vi "FTP Get File List.vi"(8 "에러 입력(에러 없음)":errorcluster, 11 "remote path":string) -> (0 "에러 출력":errorcluster, 1 "remote File path":string[](array[string]), 2 "File List":T1(array[cluster]), 4 "data":string)   [LabVIEW 2020]
uses:
  <vilib>/FTP/NI_FTP.lvlib
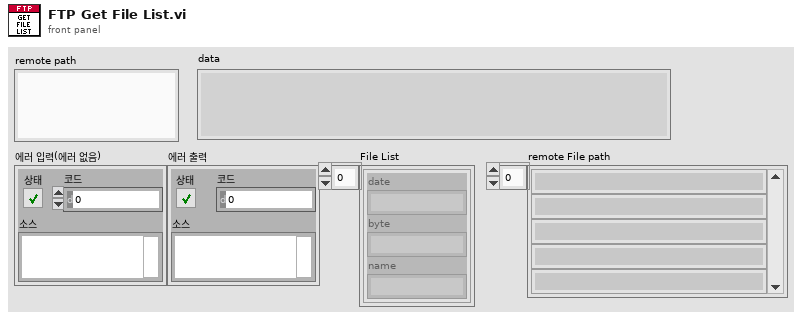
[diagram p1: front panel]
types:
  T1 = cluster{"date":string, "byte":string, "name":string}[]
  T2 = typedef "NI_FTP.lvlib/FTP Session.ctl" = refnum<k5>
  T3 = cluster{string, "trimmed string":string, "trimmed string":string}
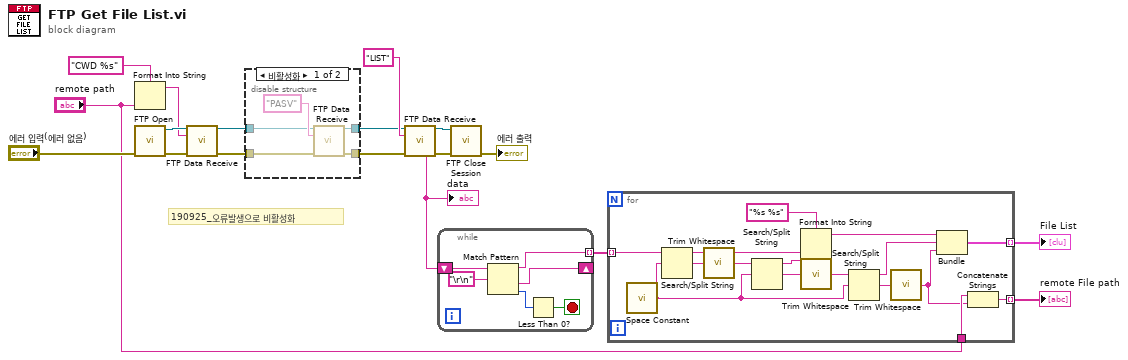
[diagram p0: block diagram]
diagram:
  # "190925_오류발생으로 비활성화"
  n1 = Format Into String(format string="CWD %s" ("포맷 문자열"), "remote path") -> (resulting string=w3:string)  [unwired: 2 in, 1 out]
  n2 = call "FTP Open.vi"("에러 입력(에러 없음)"="에러 입력(에러 없음)") -> ("에러 출력"=w7:errorcluster, "TCP 네트워크 연결 출력"=w8:T2)  [unwired: 9 in]
  n3 = call <vilib>:"FTP Data Receive.vi"("ftp session"=w8, "command"=w3, "error in (no error)"=w7) -> ("ftp session out"=w9:T2, "error out"=w10:errorcluster)  [unwired: 7 in, 4 out]
  n4 = disable-structure shown="비활성화" {
    disable-tunnel: [w23 w25] -> w13
    disable-tunnel: [w22 w24] -> w11
    disable-tunnel: w10 -> [w20 w24]
    disable-tunnel: w9 -> [w19 w25]
    frame Disabled {
      n5 = call <vilib>:"FTP Data Receive.vi"("ftp session"=w19, "command"="PASV", "error in (no error)"=w20) -> ("ftp session out"=w23:T2, "error out"=w22:errorcluster)  [unwired: 7 in, 4 out]
    }
    frame Enabled {
    }
  }
  n6 = call <vilib>:"FTP Data Receive.vi"("ftp session"=w13, "command"="LIST", "error in (no error)"=w11) -> ("ftp session out"=w14:T2, "data"=w18:string, "error out"=w12:errorcluster)  [unwired: 7 in, 3 out]
  "data" <- w18
  n7 = while {
    shift-right: [w29] -> _
    shift-left: w18 -> [w31]
    tunnel: [w28] -> w17 mode=indexing
    stop <- w26 stop-if-true
    n8 = Match Pattern(string=w31, regular expression="\r\n") -> (before substring=w28:string, after substring=w29:string, offset past match=w27:i32)  [unwired: 1 in, 1 out]
    n9 = Less Than 0?(x=w27) -> (x < 0?=w26:bool)
  }
  n10 = call <vilib>:"FTP Close Session.vi"("error in (no error)"=w12, "ftp session"=w14) -> ("error out"=→"에러 출력":errorcluster)  [unwired: 6 in, 3 out]
  n11 = for {
    tunnel: w17 -> [w47] mode=indexing
    tunnel: [w36] -> w16 mode=indexing
    tunnel: "remote path" -> [w34]
    tunnel: [w32] -> w1 mode=indexing
    n12 = call <vilib>:"Space Constant.vi"() -> ("String"=w41:string)
    n13 = Search/Split String(string=w47, search string/char (-)=w41) -> (substring before match=w40:string, match + rest of string=w46:string)  [unwired: 1 in, 1 out]
    n14 = call <vilib>:"Trim Whitespace.vi"("string"=w46) -> ("trimmed string"=w45:string)  [unwired: 1 in]
    n15 = Search/Split String(string=w45, search string/char (-)=w41) -> (substring before match=w39:string, match + rest of string=w44:string)  [unwired: 1 in, 1 out]
    n16 = Format Into String(format string="%s %s" ("포맷 문자열"), w40, w39) -> (resulting string=w35:string)  [unwired: 2 in, 1 out]
    n17 = call <vilib>:"Trim Whitespace.vi"("string"=w44) -> ("trimmed string"=w42:string)  [unwired: 1 in]
    n18 = Search/Split String(string=w42, search string/char (-)=w41) -> (substring before match=w37:string, match + rest of string=w43:string)  [unwired: 1 in, 1 out]
    n19 = call <vilib>:"Trim Whitespace.vi"("string"=w43) -> ("trimmed string"=w33:string)  [unwired: 1 in]
    n20 = Bundle(w35, "trimmed string"=w37, "trimmed string"=w33) -> (w36:T3)  [unwired: 1 in]
    n21 = Concatenate Strings(w34, w33) -> (w32:string)
  }
  "File List" <- w16
  "remote File path" <- w1
